vi "write command.vi"(8 "error in (no error)":errorcluster, 10 "string":string, 11 "BK 9202B in":refnum<class "BK 9202B.lvclass">) -> (0 "error out":errorcluster, 3 "BK 9202B out":refnum<class "BK 9202B.lvclass">)   [LabVIEW 2025, in "Power Supply.lvlib" / "BK 9202B.lvclass"]
uses:
  BK 9202B.lvclass
  BK 9202B.lvclass/BK 9202B.ctl
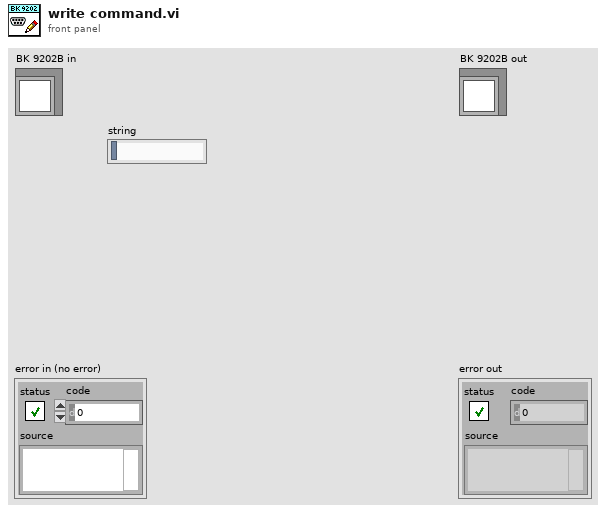
[diagram p1: front panel]
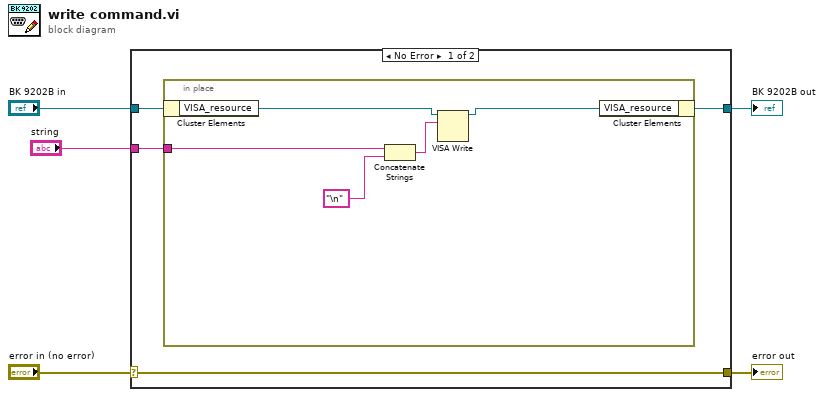
[diagram p0: block diagram]
diagram:
  n1 = case shown="No Error" "error in (no error)" {
    selector: "error in (no error)" -> [w9 w16]
    tunnel: [w9 w16] -> w4
    tunnel: [w7 w15] -> w2
    tunnel: "BK 9202B in" -> [w8 w15]
    tunnel: "string" -> [w6 _]
    frame No Error {
      n2 = in-place {
        in-place-border: w6 -> [w12]
        n3 = in-place-cluster #1(w8) -> ("VISA_resource"=w11:refnum<visa-resource-name>)
        n4 = Concatenate Strings(w12, "\n" ("string")) -> (w14:string)
        n5 = VISA Write(VISA resource name=w11, write buffer=w14) -> (VISA resource name out=w10:refnum<visa-resource-name>)  [unwired: 1 in, 2 out]
        n6 = in-place-cluster #1("VISA_resource"=w10) -> (w7:refnum<class "BK 9202B.lvclass">)
      }
    }
    frame Error {
    }
  }
  "error out" <- w4
  "BK 9202B out" <- w2
